vi "Compare Variants.vi"(8 "error in (no error)":errorcluster, 9 "Parameter 2":T1, 10 "Parameter 1":T1, 11 "Tolerant Numeric Comparator In":refnum<class "Tolerant Numeric Input Comparator.lvclass">) -> (0 "error out":errorcluster, 1 "Description":string, 2 "Equal?":bool)   [LabVIEW 2020, in "Tolerant Numeric Input Comparator.lvclass"]
uses:
  Tolerant Numeric Input Comparator.lvclass
  Tolerant Numeric Input Comparator.lvclass/Tolerant Numeric Input Comparator.ctl
  Core/Comparator/Comparator.lvclass
panel:
  in  "Numeric":dbl
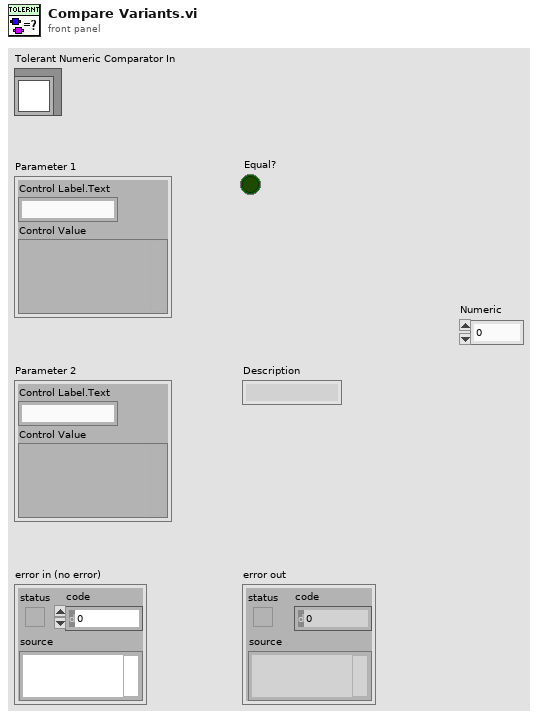
[diagram p1: front panel]
types:
  T1 = cluster{"Control Label.Text":string, "Control Value":variant}
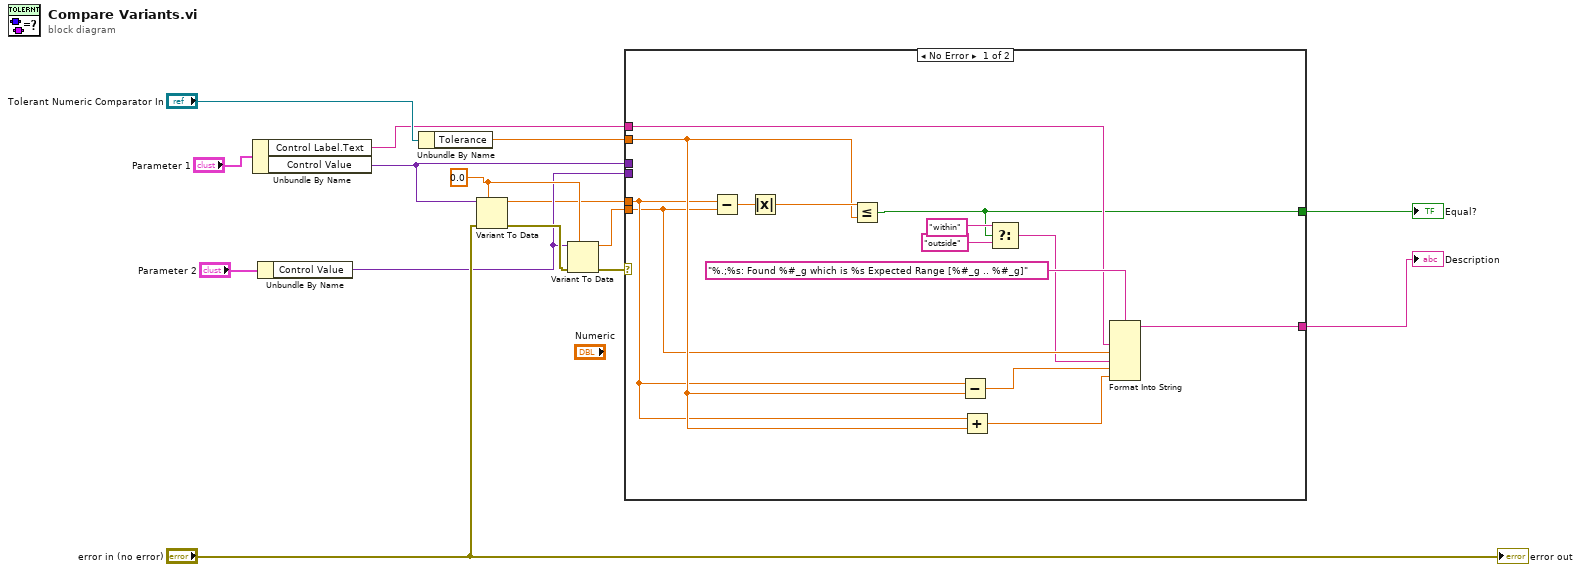
[diagram p0: block diagram]
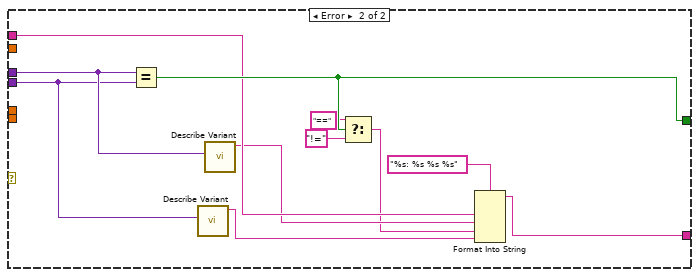
[diagram p2: hidden frame]
diagram:
  w13 = 0.0
  n1 = Unbundle By Name("Parameter 1") -> ("Control Label.Text"=w2:string, "Control Value"=w7:variant)
  n2 = Unbundle By Name("Parameter 2") -> ("Control Value"=w6:variant)
  n3 = Unbundle By Name("Tolerant Numeric Comparator In") -> ("Tolerance"=w3:dbl)
  n4 = Variant To Data(error in="error in (no error)", type=w13, Variant=w7) -> (data=w4:dbl, error out=w12:errorcluster)
  n5 = Variant To Data(error in=w12, type=w13, Variant=w6) -> (data=w5:dbl, error out=w10:errorcluster)
  n6 = case shown="No Error" w10 {
    tunnel: [w18 w39] -> w15
    tunnel: w3 -> [w26 _]
    tunnel: w4 -> [w25 _]
    tunnel: w5 -> [w22 _]
    tunnel: w7 -> [_ w40]
    tunnel: w6 -> [_ w31]
    tunnel: w2 -> [w23 w35]
    tunnel: [w21 w30] -> w1
    frame No Error {
      n7 = Subtract(x=w25, y=w22) -> (x-y=w29:dbl)
      n8 = Absolute Value(x=w29) -> (abs(x)=w28:dbl)
      n9 = Less Or Equal?(x=w28, y=w26) -> (x <= y?=w18:bool)
      n10 = Subtract(x=w25, y=w26) -> (x-y=w16:dbl)
      n11 = Add(x=w25, y=w26) -> (x+y=w27:dbl)
      n12 = Select(t="within" ("format string"), s=w18, f="outside" ("format string")) -> (s? t:f=w17:string)
      n13 = Format Into String(format string="%.;%s: Found %#_g which is %s Expected Range [%#_g .. %#_g]", w23, w22, w17, w16, w27) -> (resulting string=w21:string)  [unwired: 2 in, 1 out]
    }
    frame Error {
      n14 = Equal?(x=w40, y=w31) -> (x = y?=w39:bool)
      n15 = call "Describe Variant.vi"("Variant"=w31) -> ("Description with Type"=w32:string)  [unwired: 8 in, 2 out]
      n16 = call "Describe Variant.vi"("Variant"=w40) -> ("Description with Type"=w34:string)  [unwired: 8 in, 2 out]
      n17 = Select(t="==", s=w39, f="!=") -> (s? t:f=w33:string)
      n18 = Format Into String(format string="%s: %s %s %s", w35, w34, w33, w32) -> (resulting string=w30:string)  [unwired: 2 in, 1 out]
    }
  }
  "Equal?" <- w15
  "Description" <- w1
  "error out" <- "error in (no error)"
